vi "Start Stop All.vi"(8 "error in (no error)":errorcluster, 10 "Start? (T)":bool=TRUE, 11 "Queue in":refnum<queue>) -> (0 "error out":errorcluster, 2 "Timer Messages":string[](array[string]), 3 "Queue out":refnum<queue>)   [LabVIEW 2018, in "QueueTimer.lvlib"]
doc: "Start or stop all queue timers associated with the <b>Queue</b> reference. The <b>Timer Message</b> are returned that were started or stopped."
uses:
  QueueTimer.lvlib
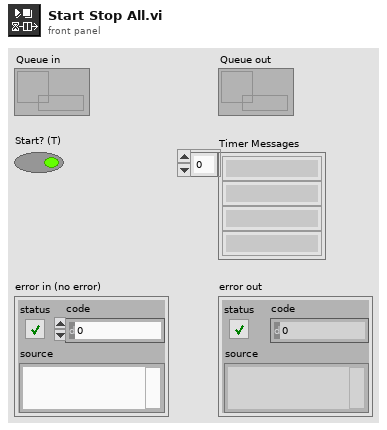
[diagram p1: front panel]
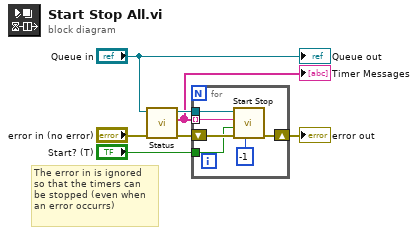
[diagram p0: block diagram]
diagram:
  # "The error in is ignored\nso that the timers can\nbe stopped (even when\nan error occurrs)"
  n1 = call "Status.vi"("error in (no error)"="error in (no error)", "Queue in"="Queue in") -> ("error out"=w2:errorcluster, "Timer Messages"=w1:string[], "Queue out"=w4:refnum<queue>)  [unwired: 4 in, 3 out]
  "Timer Messages" <- w1
  n2 = for {
    tunnel: "Start? (T)" -> [w10]
    shift-right: [w8] -> w7
    shift-left: w2 -> [w13]
    tunnel: w4 -> [w12]
    tunnel: w1 -> [w11] mode=indexing
    n3 = call "Start Stop.vi"("ms Delay (-1=No change)"=-1, "error in (no error)"=w13, "Start? (T)"=w10, "Timer Message"=w11, "Queue in"=w12) -> ("error out"=w8:errorcluster)  [unwired: 5 in, 1 out]
  }
  "error out" <- w7
  "Queue out" <- "Queue in"
